vi "Instrument.Temperhum.AppLauncher.vi"(8 "error in":errorcluster, 10 "Config Window":bool, 11 "Debug Mode":bool) -> (0 "error out":errorcluster)   [LabVIEW 2019, in "Instrument.Temperhum.lvclass"]
uses:
  Instrument.Temperhum.lvclass
  <vilib>/JKI/JKI SMO/SMO/Typedefs/SMOState --Enum.ctl
  Instrument UI.Temperhum/Typedefs/Type--enum.ctl
  <userlib>/LevyLab/Instrument Framework/SMOs/Instrument/Instrument.lvclass
  C:/Program Files (x86)/National Instruments/LabVIEW 2019/vi.lib/JKI/JKI SMO/SMO/SMO.lvclass
  <userlib>/LevyLab/Instrument Framework/SMOs/Instrument UI/Instrument UI.lvclass
  C:/Program Files (x86)/National Instruments/LabVIEW 2019/vi.lib/JKI/JKI SMO/SMO.UI/SMO.UI.lvclass
  Instrument UI.Temperhum/Instrument UI.Temperhum.lvclass
  C:/Program Files (x86)/National Instruments/LabVIEW 2019/user.lib/LevyLab/Instrument Framework/SMOs/Instrument UI/Instrument UI.lvclass
  C:/Program Files (x86)/National Instruments/LabVIEW 2019/user.lib/LevyLab/Instrument Framework/SMOs/Instrument/Instrument.lvclass
  <userlib>/LevyLab/Instrument Framework/SMOs/Configuration/Configuration.lvclass
  <vilib>/JKI/JKI SMO/SMO/SMO.lvclass/SMO.ctl
  <userlib>/LevyLab/Instrument Framework/SMOs/Configuration/Configuration.lvclass/Configuration.ctl
  Instrument UI.Temperhum/Typedefs/Instrument UI.Temperhum.UI--Cluster.ctl
  Temperhum.PCSensor/Temperhum.PCSensor.lvclass
  Temperhum.Thorlabs/Temperhum.Thorlabs.lvclass
  <vilib>/JKI/JKI SMO/SMO/Private/ReftoDVR--SMO.vi
  <vilib>/JKI/JKI SMO/SMO/SMO.lvclass
  <vilib>/JKI/JKI SMO/SMO.UI/SMO.UI.lvclass
panel:
  in  "Examine Configuration.ini":bool
  in  "Choose hardware type":T1
  in  "Splash Status":string="Push Start to Start..." caption="String"
  in  "Start Application":bool caption="Play"
  in  "Stop Application":bool caption="Stop"
  out "UI SMO State":T2=enum."Stopped"
  out "SMO State":T2
  # "Example Instrument SMO Test Launcher"
  # "For instructions on how to use the JKI State Machine Objects, examples and video tutorials, visit:\nhttp://jki.net/state-machine-objects/\n\nJKI State Machine Objects™\nhttp://jki.net/state-machine-objects/\nCopyright (C) 2005-2015, JKI <info@jki.net>\nALL RIGHTS RESERVED"
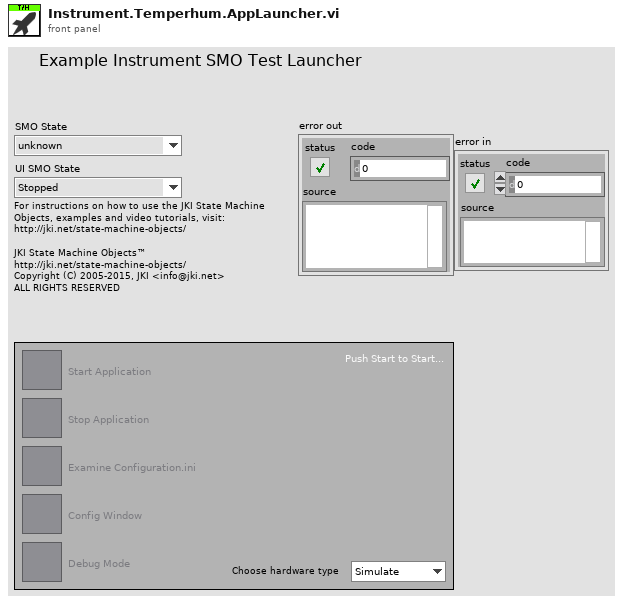
[diagram p1: front panel]
types:
  T1 = typedef "Instrument UI.Temperhum.lvclass/Type--enum.ctl" = enum16{"Simulate", "PCsensor", "Thorlabs"}
  T2 = typedef "SMO.lvclass/SMOState --Enum.ctl" = enum16{"unknown", "Created", "Started", "Stopped"}
  T3 = enum32{"Invalid", "Standard", "Closed", "Hidden", "Minimized", "Maximized"}
  T4 = enum32{"invalid app kind", "Development System", "Run Time System", "Student Edition", "Embedded LabVIEW", "Evaluation", "Custom"}
  T5 = typedef "Instrument UI.Temperhum.lvclass/Instrument UI.Temperhum.UI--Cluster.ctl" = cluster{"HW Type":T1}
  T6 = cluster{"Core":cluster{"Current VI Reference":refnum<vi>, "Close Panel on Exit?":bool}, "Instrument":refnum<class "Instrument.lvclass">, "Instrument UI":refnum<class "Instrument UI.lvclass">, "Configuration":refnum<class "Configuration.lvclass">}
  T7 = cluster{"Current VI Reference":refnum<vi>, "Close Panel on Exit?":bool}
  T8 = typedef "SMO.lvclass/Public Events.ctl" = cluster{"Error":refnum<user-event>, "State":refnum<user-event>, "Reserve State":refnum<user-event>}
  T9 = cluster{"Event Registration Refnum":refnum<event-registration>, "Event Registration Refnum":refnum<event-registration>}
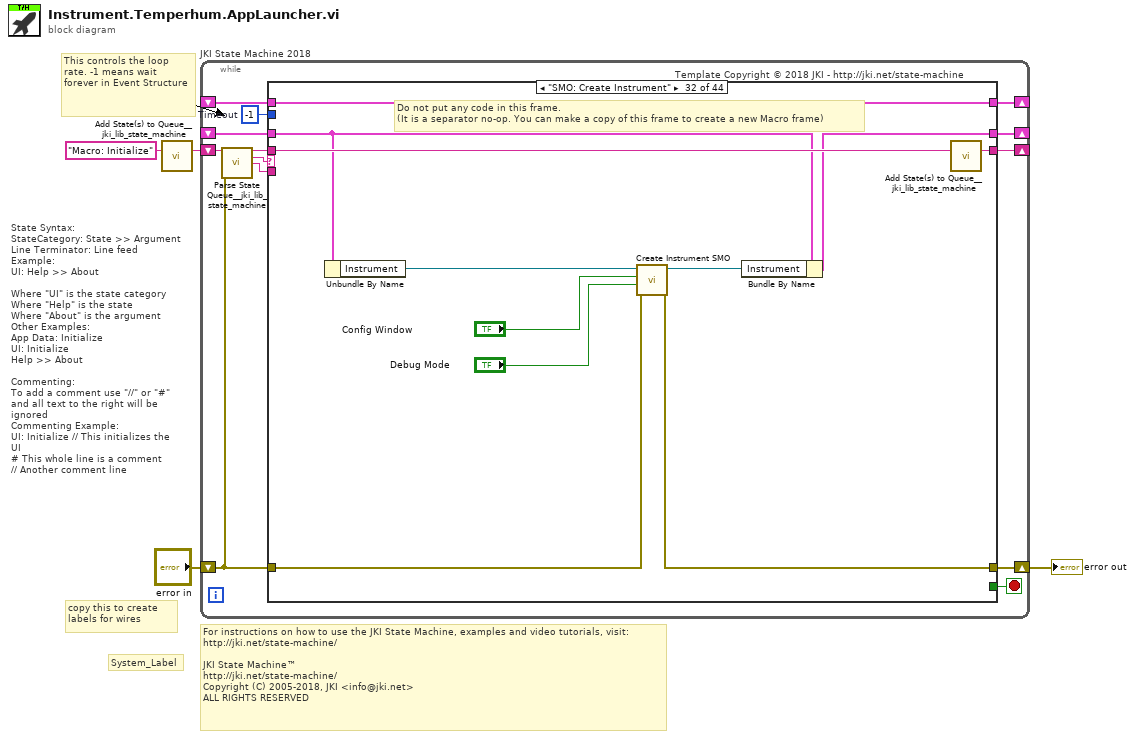
[diagram p0: block diagram]
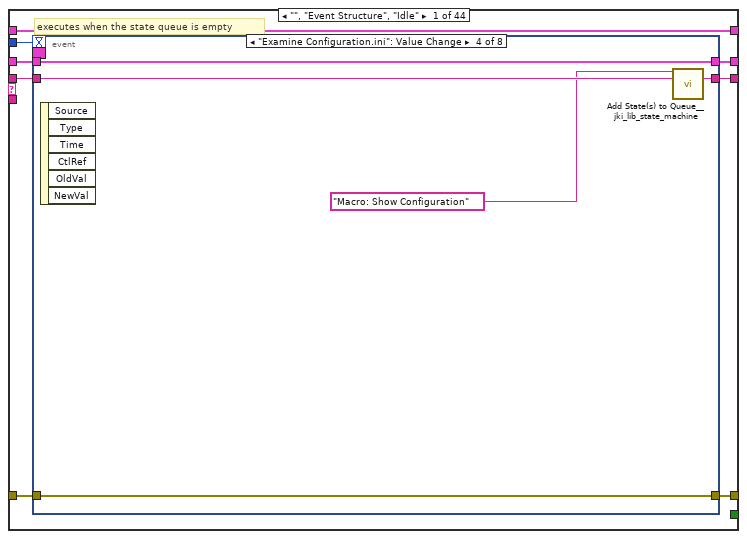
[diagram p2: hidden frame]
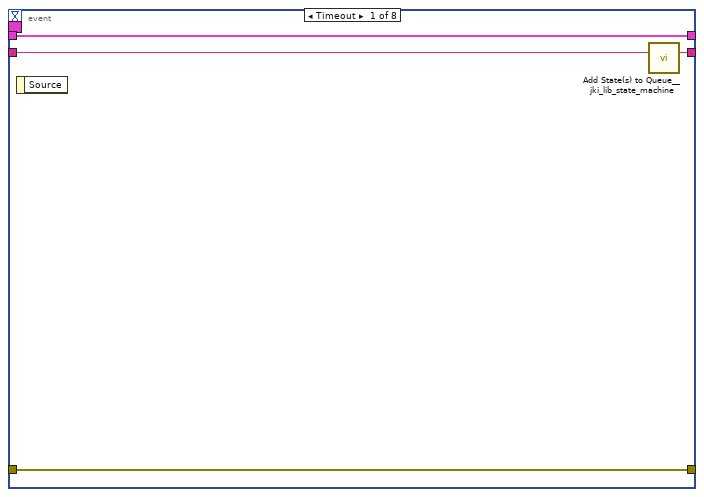
[diagram p3: hidden frame]
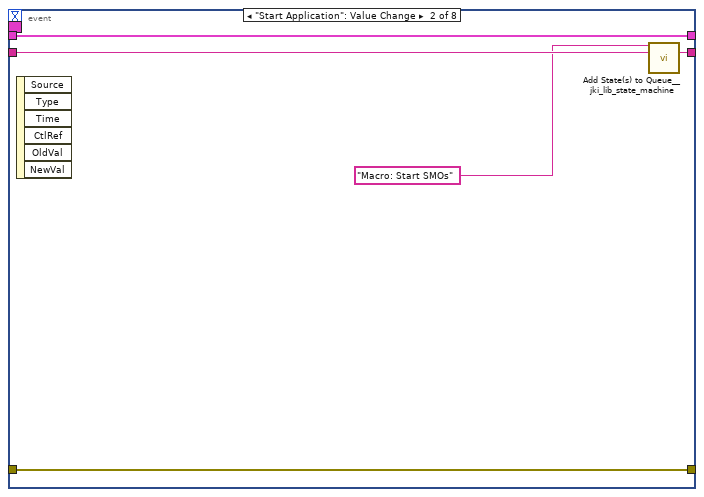
[diagram p4: hidden frame]
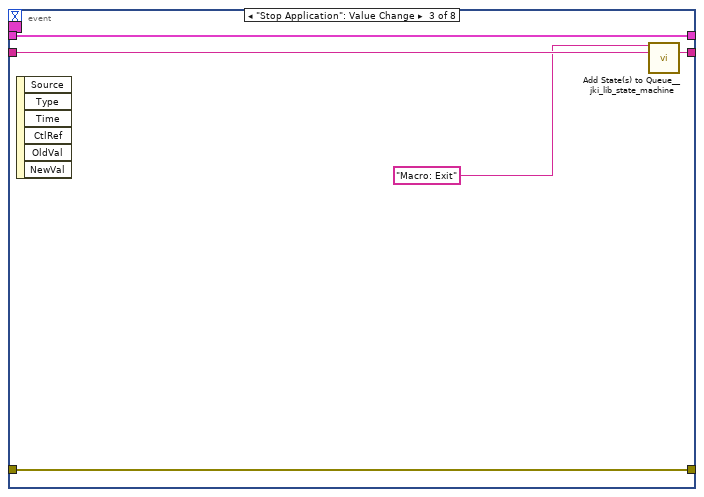
[diagram p5: hidden frame]
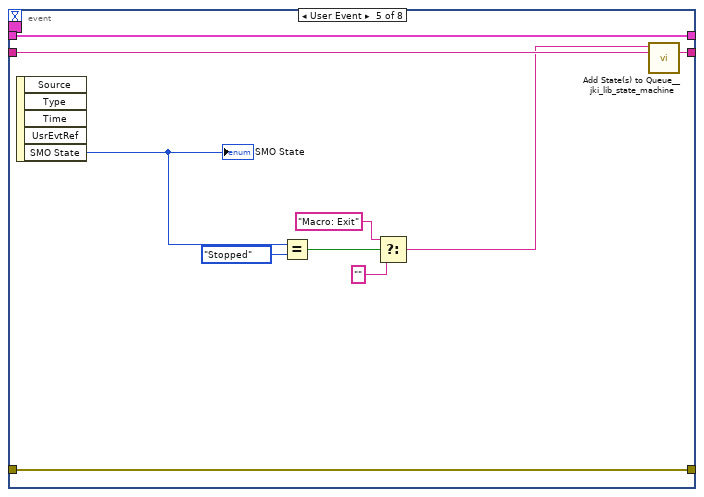
[diagram p6: hidden frame]
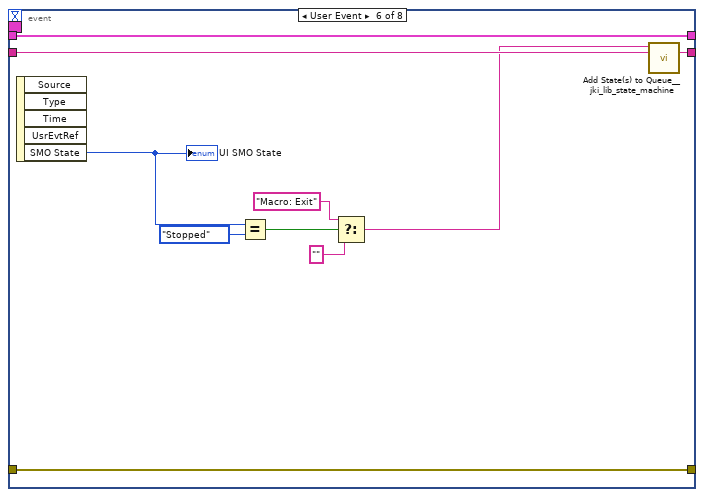
[diagram p7: hidden frame]
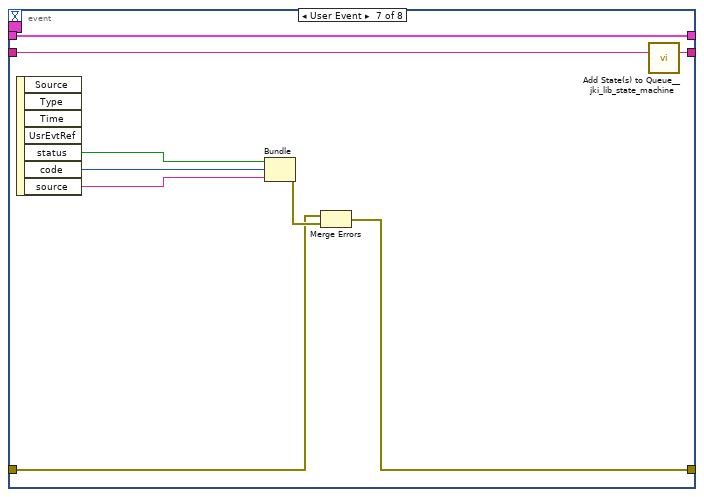
[diagram p8: hidden frame]
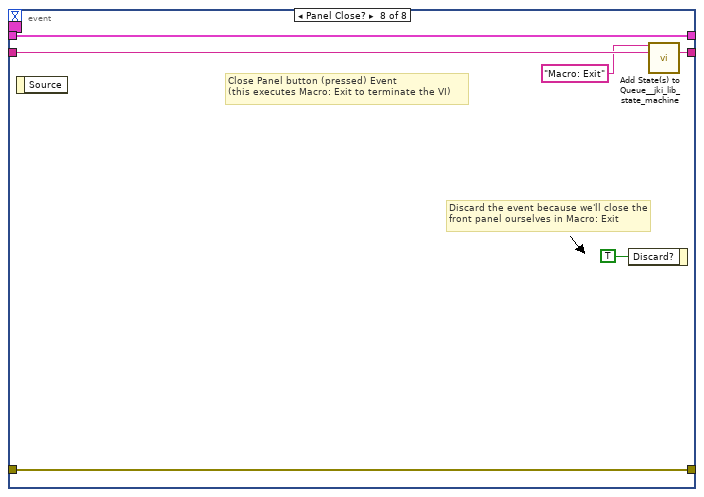
[diagram p9: hidden frame]
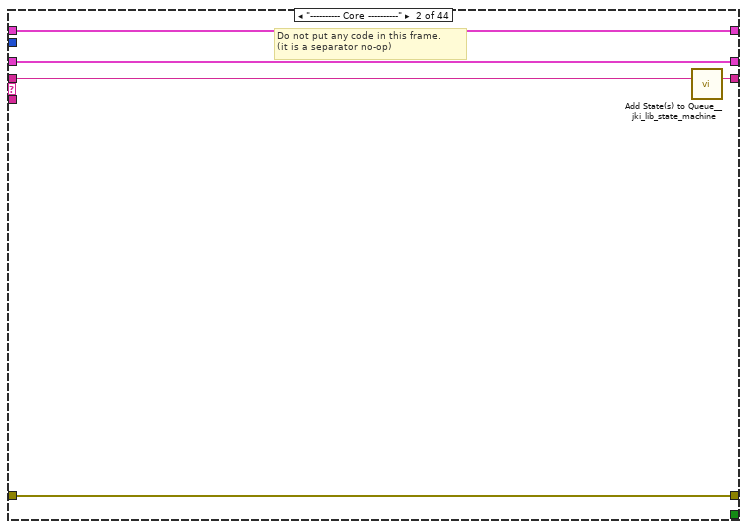
[diagram p10: hidden frame]
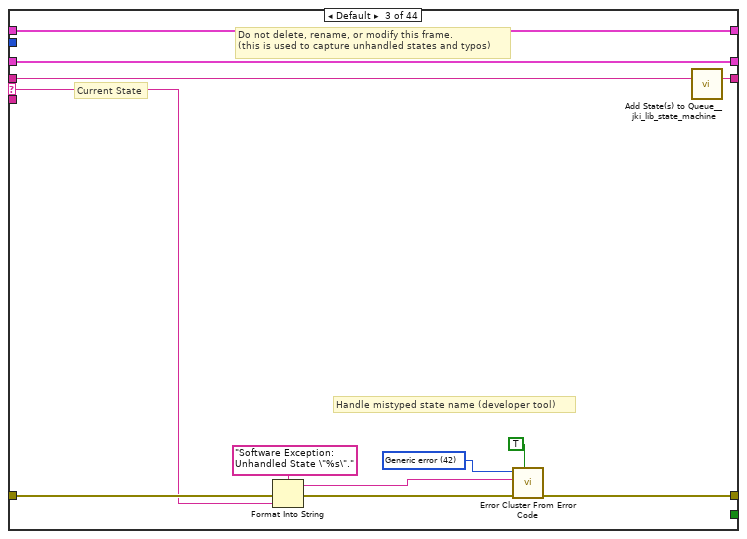
[diagram p11: hidden frame]
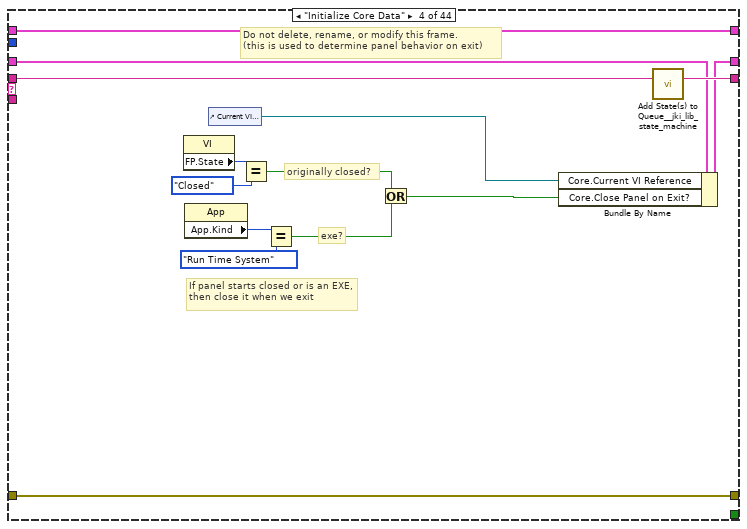
[diagram p12: hidden frame]
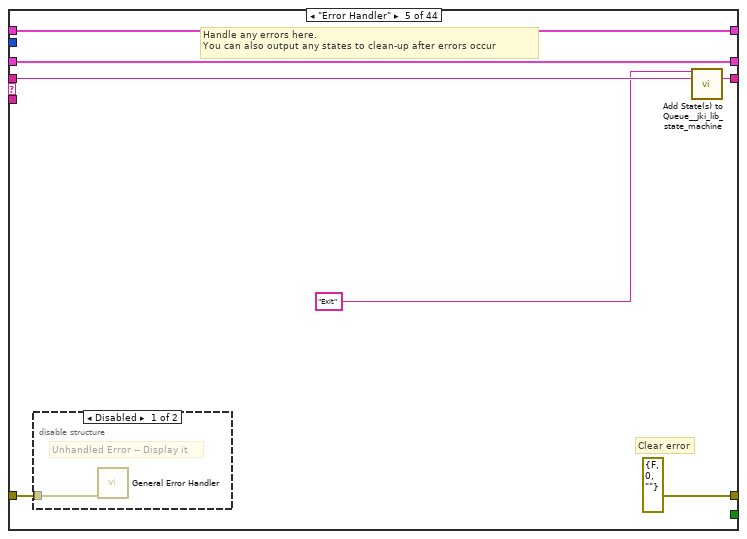
[diagram p13: hidden frame]
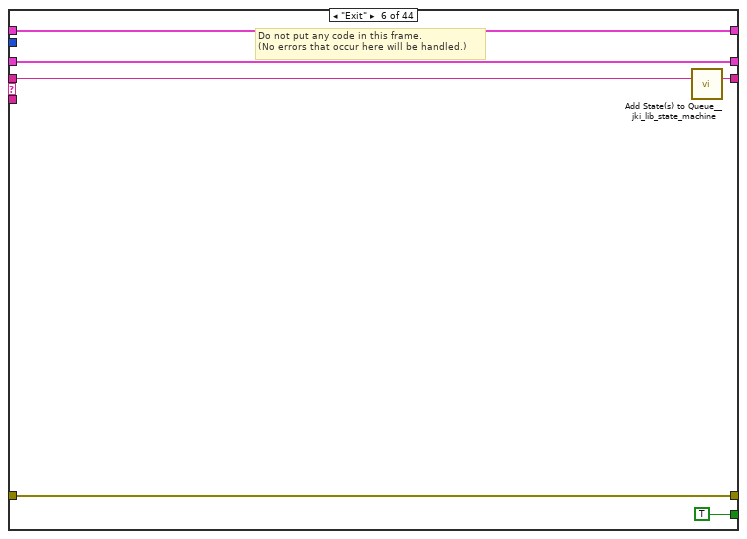
[diagram p15: hidden frame]
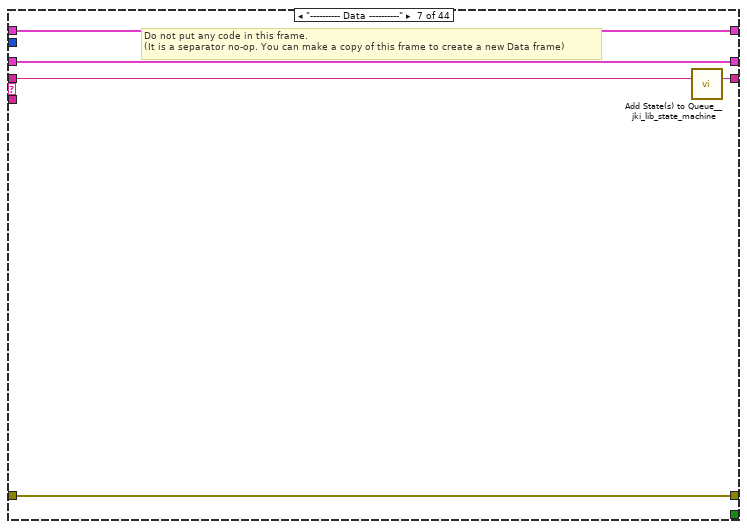
[diagram p16: hidden frame]
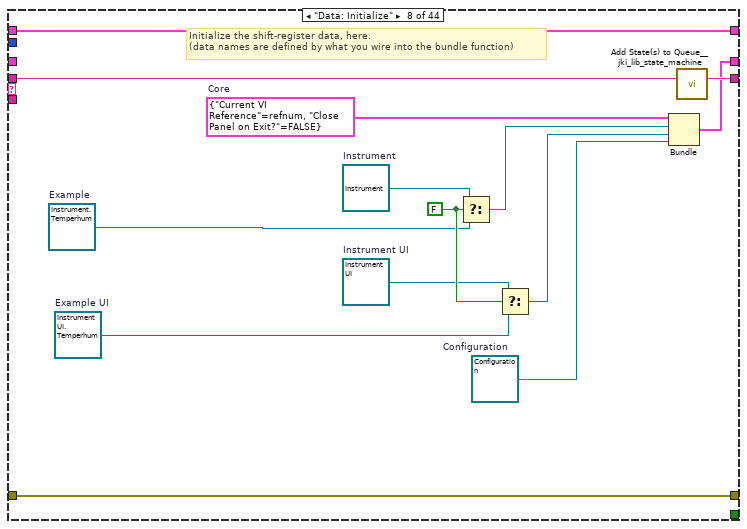
[diagram p17: hidden frame]
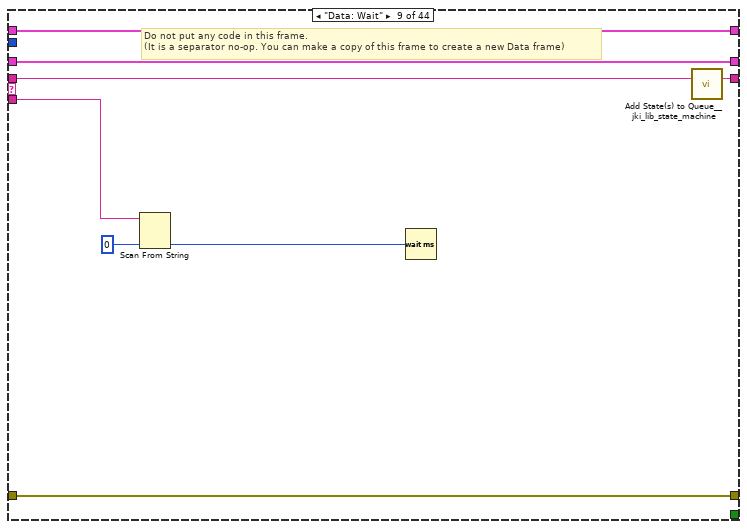
[diagram p18: hidden frame]
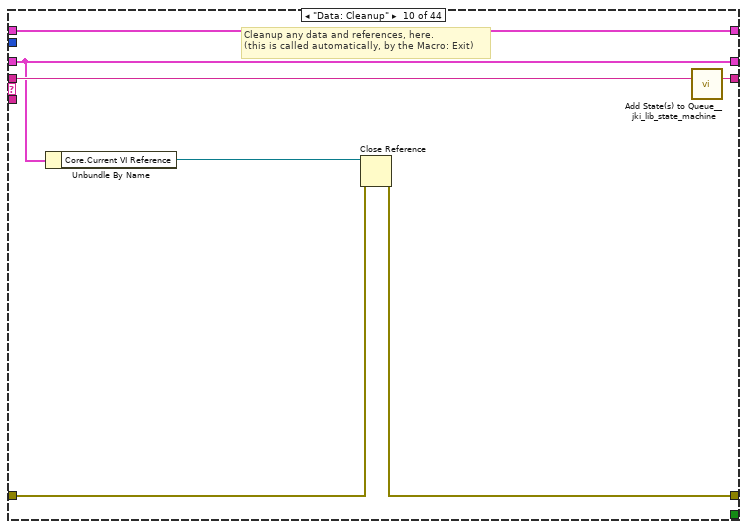
[diagram p19: hidden frame]
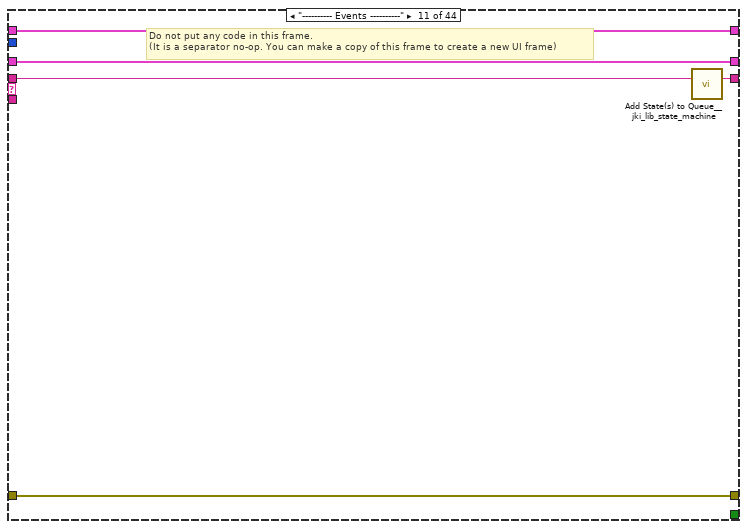
[diagram p20: hidden frame]
diagram:
  # "For instructions on how to use the JKI State Machine, examples and video tutorials, visit:\nhttp://jki.net/state-machine/\n\nJKI State Machine™\nhttp://jki.net/state-machine/\nCopyright (C) 2005-2018, JKI <info@jki.net>\nALL RIGHTS RESERVED"
  # "State Syntax:\nStateCategory: State >> Argument\nLine Terminator: Line feed\nExample:\nUI: Help >> About\n\nWhere \"UI\" is the state category\nWhere \"Help\" is the state\nWhere \"About\" is the argument\nOther Examples:\nApp Data: Initialize\nUI: Initialize\nHelp >> About\n\nCommenting:\nTo add a comment use \"//\" or \"#\" and all text to the right will be ignored\nCommenting Example:\nUI: Initialize // This initializes the UI\n# This whole line is a comment\n// Another comment line"
  # "copy this to create labels for wires"
  # "This controls the loop rate. -1 means wait forever in Event Structure"
  # "System_Label"
  n1 = call <vilib>:"Add State(s) to Queue__jki_lib_state_machine.vi"("State(s) in (\"\")"="Macro: Initialize") -> ("States Out"=w4:string)  [unwired: 14 in]
  n2 = while "JKI State Machine 2018" {
    shift-right: [w11] -> _
    shift-left: _ -> [w6]
    shift-right: [w14] -> w2
    shift-left: "error in" -> [w9]
    shift-right: [w13] -> _
    shift-left: w4 -> [w15]
    shift-right: [w8] -> _
    shift-left: _ -> [w7]
    stop <- w12 stop-if-true
    w10 = -1  # Timeout
    # "Template Copyright © 2018 JKI - http://jki.net/state-machine"
    n3 = call <vilib>:"Parse State Queue__jki_lib_state_machine.vi"("State Queue"=w15, "Error In (no error)"=w9) -> ("Remaining States"=w17:string, "Current State"=w5:string, "Arguments"=w16:string)  [unwired: 11 in]
    n4 = case shown="\"SMO: Create Instrument\"" w5 {
      selector: w5 -> [_ _ w86 _ _ _ _ _ _ _ _ _ _ _ _ _ _ _ _ _ _ _ _ _ _ _ _ _ _ _ _ _ _ _ _ _ _ _ _ _ _ _ _ _]
      tunnel: w17 -> [w25 w84 w90 w110 w117 w124 w129 w143 w151 w158 w163 w176 w182 w187 w193 w200 w212 w290 w297 w309 w321 w335 w340 w345 w351 w357 w363 w369 w381 w386 w395 w409 w418 w428 w435 w446 w461 w476 w491 w506 w521 w530 w537 w542]
      tunnel: w16 -> [_ _ _ _ _ _ _ _ w144 _ _ _ _ _ _ w195 w206 _ _ _ _ _ _ _ _ _ _ _ _ _ _ _ _ _ _ _ _ _ _ _ _ _ w534 _]
      tunnel: [w22 w82 w92 w107 errorcluster {"status"=FALSE, "code"=0, "source"=""} ("error out") w121 w127 w138 w149 w154 w161 w165 w177 w185 w188 w196 w209 w280 w292 w302 w314 w326 w338 w343 w349 w355 w361 w367 w379 w384 w393 w405 w410 w419 w429 w442 w457 w472 w488 w503 w518 w528 w532 w540] -> w14
      tunnel: w9 -> [w21 w82 w91 w107 w113 w121 w127 w138 w149 w155 w161 w167 w178 w185 w190 w197 w210 w281 w291 w301 w313 w322 w338 w343 w349 w355 w361 w367 w379 w384 w393 w406 w411 w420 w430 w439 w453 w469 w486 w501 w514 w528 w533 w540]
      tunnel: [w24 w83 w89 w109 w116 w123 w128 w142 w150 w157 w162 w175 w181 w186 w192 w199 w211 w289 w296 w308 w320 w334 w339 w344 w350 w356 w362 w368 w380 w385 w394 w408 w417 w427 w434 w445 w460 w475 w490 w505 w520 w529 w536 w541] -> w13
      tunnel: [_ _ _ _ _ TRUE _ _ _ _ _ _ _ _ _ _ _ _ _ _ _ _ _ _ _ _ _ _ _ _ _ _ _ _ _ _ _ _ _ _ _ _ _ _] -> w12
      tunnel: [w20 w81 w88 w108 w114 w122 w126 w141 w148 w153 w160 w170 w180 w184 w191 w198 w208 w278 w293 w299 w316 w330 w337 w342 w348 w354 w360 w366 w378 w383 w388 w404 w413 w424 w432 w443 w458 w473 w487 w502 w517 w527 w535 w539] -> w11
      tunnel: w10 -> [w19 _ _ _ _ _ _ _ _ _ _ _ _ _ _ _ _ _ _ _ _ _ _ _ _ _ _ _ _ _ _ _ _ _ _ _ _ _ _ _ _ _ _ _]
      tunnel: [w18 w80 w85 w97 w111 w119 w125 w139 w147 w152 w159 w173 w179 w183 w189 w194 w205 w279 w295 w307 w319 w333 w336 w341 w346 w353 w359 w365 w372 w382 w392 w407 w416 w426 w433 w444 w459 w474 w489 w504 w519 w526 w531 w538] -> w8
      tunnel: w7 -> [w18 w80 w85 w97 w111 w119 w125 w139 w147 w152 w159 _ w179 w183 w189 w194 w205 w279 w295 w307 w319 w333 w336 w341 w346 w353 w359 w365 w372 w382 w392 w407 w416 w426 w433 w444 w459 w474 w489 w504 w519 w526 w531 w538]
      tunnel: w6 -> [w23 w81 w88 w103 w114 w122 w126 _ w148 w153 w160 w170 w180 w184 w191 w198 w208 w278 w293 w298 w315 w329 w337 w342 w348 w354 w360 w366 w378 w383 w389 w402 w414 w425 w432 w443 w458 w473 w487 w502 w517 w527 w535 w539]
      frame "", "Event Structure", "Idle" {
        # "executes when the state queue is empty"
        n5 = event shown="[3] \"Examine Configuration.ini\": Value Change" {
          selector: w18 -> [_ _ _ _ _ _ _ _]
          dyn-events: _ -> [_ _ _ _ _ _ _ _]
          timeout: w19 -> [_ _ _ _ _ _ _ _]
          tunnel: w25 -> [w29 w34 w39 w44 w54 w64 w73 w79]
          tunnel: [w28 w33 w38 w43 w53 w63 w72 w78] -> w24
          tunnel: w23 -> [w26 w31 w36 w41 w51 w61 w71 w76]
          tunnel: [w27 w32 w37 w42 w52 w62 w68 w77] -> w22
          tunnel: w21 -> [w27 w32 w37 w42 w52 w62 w69 w77]
          tunnel: [w26 w31 w36 w41 w51 w61 w71 w76] -> w20
          event Timeout {
            n6 = event-data() -> ()  [unwired: 1 in, 1 out]
            n7 = call <vilib>:"Add State(s) to Queue__jki_lib_state_machine.vi"("State(s) in (\"\")"=w29) -> ("States Out"=w28:string)  [unwired: 14 in]
          }
          event "Start Application": Value Change {
            n8 = event-data() -> ()  [unwired: 1 in, 6 out]
            n9 = call <vilib>:"Add State(s) to Queue__jki_lib_state_machine.vi"("State(s) in Front (\"\")"="Macro: Start SMOs" ("State(s) in Front (\"\")"), "State(s) in (\"\")"=w34) -> ("States Out"=w33:string)  [unwired: 13 in]
          }
          event "Stop Application": Value Change {
            n10 = event-data() -> ()  [unwired: 1 in, 6 out]
            n11 = call <vilib>:"Add State(s) to Queue__jki_lib_state_machine.vi"("State(s) in Front (\"\")"="Macro: Exit" ("State(s) in Front (\"\")"), "State(s) in (\"\")"=w39) -> ("States Out"=w38:string)  [unwired: 13 in]
          }
          event "Examine Configuration.ini": Value Change {
            n12 = event-data() -> ()  [unwired: 1 in, 6 out]
            n13 = call <vilib>:"Add State(s) to Queue__jki_lib_state_machine.vi"("State(s) in Front (\"\")"="Macro: Show Configuration" ("State(s) in Front (\"\")"), "State(s) in (\"\")"=w44) -> ("States Out"=w43:string)  [unwired: 13 in]
          }
          event User Event {
            n14 = event-data() -> ("SMO State"=w46:T2)  [unwired: 1 in, 4 out]
            "SMO State" <- w46
            n15 = Equal?(x=w46, y=SMOState_--Enum."Stopped") -> (x = y?=w49:bool)
            n16 = Select(t="Macro: Exit", s=w49, f="" ("State(s) in Front (\"\")")) -> (s? t:f=w45:string)
            n17 = call <vilib>:"Add State(s) to Queue__jki_lib_state_machine.vi"("State(s) in Front (\"\")"=w45, "State(s) in (\"\")"=w54) -> ("States Out"=w53:string)  [unwired: 13 in]
          }
          event User Event {
            n18 = event-data() -> ("SMO State"=w55:T2)  [unwired: 1 in, 4 out]
            "UI SMO State" <- w55
            n19 = Equal?(x=w55, y=SMOState_--Enum."Stopped") -> (x = y?=w59:bool)
            n20 = Select(t="Macro: Exit", s=w59, f="" ("State(s) in Front (\"\")")) -> (s? t:f=w57:string)
            n21 = call <vilib>:"Add State(s) to Queue__jki_lib_state_machine.vi"("State(s) in Front (\"\")"=w57, "State(s) in (\"\")"=w64) -> ("States Out"=w63:string)  [unwired: 13 in]
          }
          event User Event {
            n22 = event-data() -> ("status"=w65:bool, "code"=w67:i32, "source"=w66:string)  [unwired: 1 in, 4 out]
            n23 = Bundle("status"=w65, "code"=w67, "source"=w66) -> (w70:errorcluster)  [unwired: 1 in]
            n24 = Merge Errors(w69, w70) -> (w68:errorcluster)
            n25 = call <vilib>:"Add State(s) to Queue__jki_lib_state_machine.vi"("State(s) in (\"\")"=w73) -> ("States Out"=w72:string)  [unwired: 14 in]
          }
          event Panel Close? {
            # "Discard the event because we'll close the front panel ourselves in Macro: Exit"
            # "Close Panel button (pressed) Event\n(this executes Macro: Exit to terminate the VI)"
            n26 = event-data() -> ()  [unwired: 1 in, 1 out]
            n27 = event-data("Discard?"=TRUE) -> ()  [unwired: 1 in, 1 out]
            n28 = call <vilib>:"Add State(s) to Queue__jki_lib_state_machine.vi"("State(s) in Front (\"\")"="Macro: Exit", "State(s) in (\"\")"=w79) -> ("States Out"=w78:string)  [unwired: 13 in]
          }
        }
      }
      frame "---------- Core ----------" {
        # "Do not put any code in this frame.\n(it is a separator no-op)"
        n29 = call <vilib>:"Add State(s) to Queue__jki_lib_state_machine.vi"("State(s) in (\"\")"=w84) -> ("States Out"=w83:string)  [unwired: 14 in]
      }
      frame Default {
        w95 = 42 items=["No error", "Argument error", "Memory is full", "Out of zone", "End of file", "File already open", "Generic file I/O error", "File not found", "File permission error", "Disk is full", "Duplicate path", "Too many files open", "System feature not enabled", "Resource file not found", "Cannot add resource", "Resource not found", "Image not found", "Image memory error", "Pen does not exist", "Config type invalid", "Config token not found", "Config parse error", "Config memory error", "Bad external code format", "Bad external code offset", "External code not present", "Null window", "Destroy window error", "Null menu", "Print aborted", "Bad print record", "Print driver error", "Windows error during printing", "Memory error during printing", "Print dialog error", "Generic print error", "Invalid device refnum", "Device not found", "Device parameter error", "Device unit error", "Cannot open device", "Device call aborted", "Generic error", "Cancelled by user", "Object ID too low", "Object ID too high", "Object not in heap", "Unknown heap", "Unknown object (invalid DefProc)", "Unknown object (DefProc not in table)", "Message out of range", "Invalid (null) method", "Unknown message", "Manager call not supported", "Bad address", "Network operation in progress", "Network operation timed out", "Connection is busy", "Network attribute not supported", "Network error", "Address in use", "System out of memory", "Connection aborted", "Connection refused", "Not connected", "Already connected", "Connection closed", "Initialization error (interapplication manager)", "Bad occurrence", "Wait on unbound occurrence handler", "Occurrence queue overflow", "Datalog type conflict", "Unused", "Unrecognized type (interapplication manager)", "Memory corrupt", "Failed to make temporary DLL", "Old CIN version", "Drag socket not found", "Failed to load drop-object", "Failed to register OLE object", "Failed to release OLE object", "Format specifier type mismatch", "Unknown format specifier", "Too few format specifiers", "Too many format specifiers", "Scan failed", "Newer CIN version", "Error converting to variant", "Runtime menu error", "Password tampered", "Variant attribute not found", "Incompatible variant data type", "Event data is not available", "Event Store is not present", "Occurrence is not found", "Event Queue is not created", "Event info is not available", "Refnum passed is NULL", "Error retrieving Class GUID", "Error retrieving CoClass GUID", "Error retrieving TypeLib GUID.", "Bad built application magic bytes.", "Specific driver is different from the specific driver associated with the Logical Name.", "There is no session opened to the class driver.", "Max Error", "MAX - Error with config objects", "MAX - Error loading configuration", "MAX - Group not supported"]
        # "Current State"
        # "Do not delete, rename, or modify this frame.\n(this is used to capture unhandled states and typos)"
        # "Handle mistyped state name (developer tool)"
        n30 = Format Into String(format string="Software Exception: Unhandled State \"%s\"." ("message"), error in=w91, w86) -> (resulting string=w94:string, error out=w93:errorcluster)  [unwired: 1 in]
        n31 = call <vilib>:"Error Cluster From Error Code.vi"("show call chain? (False)"=TRUE, "error in (no error)"=w93, "error message (\"\")"=w94, "error code (0)"=w95) -> ("error out"=w92:errorcluster)  [unwired: 5 in]
        n32 = call <vilib>:"Add State(s) to Queue__jki_lib_state_machine.vi"("State(s) in (\"\")"=w90) -> ("States Out"=w89:string)  [unwired: 14 in]
      }
      frame "Initialize Core Data" {
        # "Do not delete, rename, or modify this frame.\n(this is used to determine panel behavior on exit)"
        # "originally closed?"
        # "exe?"
        # "If panel starts closed or is an EXE, then close it when we exit"
        n33 = property class="VI"() -> ("FP.State"=w100:T3)  [unwired: 2 in, 2 out]
        n34 = property class="App"() -> ("App.Kind"=w106:T4)  [unwired: 2 in, 2 out]
        n35 = control-ref of="Current VI Reference"() -> (w101:refnum<vi>)
        n36 = Equal?(x=w100, y=T3."Closed" ("Front Panel Window:State")) -> (x = y?=w98:bool)
        n37 = Equal?(x=w106, y=T4."Run Time System" ("Application:Kind")) -> (x = y?=w104:bool)
        n38 = Or(x=w98, y=w104) -> (x .or. y?=w102:bool)
        n39 = Bundle By Name(cluster=w103, "Core.Current VI Reference"=w101, "Core.Close Panel on Exit?"=w102) -> (w108:T6)
        n40 = call <vilib>:"Add State(s) to Queue__jki_lib_state_machine.vi"("State(s) in (\"\")"=w110) -> ("States Out"=w109:string)  [unwired: 14 in]
      }
      frame "Error Handler" {
        # "Handle any errors here.\nYou can also output any states to clean-up after errors occur"
        # "Clear error"
        n41 = disable-structure shown="Disabled" {
          disable-tunnel: w113 -> [w118 _]
          frame Disabled {
            # "Unhandled Error -- Display it"
            n42 = call <vilib>:"General Error Handler.vi"("error in (no error)"=w118) -> ()  [unwired: 10 in, 5 out]
          }
          frame Enabled {
          }
        }
        n43 = call <vilib>:"Add State(s) to Queue__jki_lib_state_machine.vi"("State(s) in Front (\"\")"="Exit", "State(s) in (\"\")"=w117) -> ("States Out"=w116:string)  [unwired: 13 in]
      }
      frame "Exit" {
        # "Do not put any code in this frame.\n(No errors that occur here will be handled.)"
        n44 = call <vilib>:"Add State(s) to Queue__jki_lib_state_machine.vi"("State(s) in (\"\")"=w124) -> ("States Out"=w123:string)  [unwired: 14 in]
      }
      frame "---------- Data ----------" {
        # "Do not put any code in this frame.\n(It is a separator no-op. You can make a copy of this frame to create a new Data frame)"
        n45 = call <vilib>:"Add State(s) to Queue__jki_lib_state_machine.vi"("State(s) in (\"\")"=w129) -> ("States Out"=w128:string)  [unwired: 14 in]
      }
      frame "Data: Initialize" {
        w130 = refnum<class "Configuration.lvclass"> refnum  # Configuration
        w134 = FALSE ("s")
        w133 = refnum<class "Instrument.Temperhum.lvclass"> refnum  # Example
        w132 = refnum<class "Instrument UI.Temperhum.lvclass"> refnum  # Example UI
        w131 = refnum<class "Instrument UI.lvclass"> refnum  # Instrument UI
        w137 = refnum<class "Instrument.lvclass"> refnum  # Instrument
        w140 = T7 {"Current VI Reference"=refnum, "Close Panel on Exit?"=FALSE}  # Core
        # "Initialize the shift-register data, here.\n(data names are defined by what you wire into the bundle function)"
        n46 = Select(t=w137, s=w134, f=w133) -> (s? t:f=w136:refnum<class "Instrument.lvclass">)
        n47 = Select(t=w131, s=w134, f=w132) -> (s? t:f=w135:refnum<class "Instrument UI.lvclass">)
        n48 = Bundle("Core"=w140, "Instrument"=w136, "Instrument UI"=w135, "Configuration"=w130) -> (w141:T6)  [unwired: 1 in]
        n49 = call <vilib>:"Add State(s) to Queue__jki_lib_state_machine.vi"("State(s) in (\"\")"=w143) -> ("States Out"=w142:string)  [unwired: 14 in]
      }
      frame "Data: Wait" {
        # "Do not put any code in this frame.\n(It is a separator no-op. You can make a copy of this frame to create a new Data frame)"
        n50 = Scan From String(input string=w144, default 1=u32 0) -> (output 1=w145:u32)  [unwired: 3 in, 3 out]
        n51 = Wait (ms)(milliseconds to wait=w145) -> ()  [unwired: 1 out]
        n52 = call <vilib>:"Add State(s) to Queue__jki_lib_state_machine.vi"("State(s) in (\"\")"=w151) -> ("States Out"=w150:string)  [unwired: 14 in]
      }
      frame "Data: Cleanup" {
        # "Cleanup any data and references, here.\n(this is called automatically, by the Macro: Exit)"
        n53 = Unbundle By Name(w153) -> ("Core.Current VI Reference"=w156:refnum<vi>)
        n54 = Close Reference(reference=w156, error in (no error)=w155) -> (error out=w154:errorcluster)
        n55 = call <vilib>:"Add State(s) to Queue__jki_lib_state_machine.vi"("State(s) in (\"\")"=w158) -> ("States Out"=w157:string)  [unwired: 14 in]
      }
      frame "---------- Events ----------" {
        # "Do not put any code in this frame.\n(It is a separator no-op. You can make a copy of this frame to create a new UI frame)"
        n56 = call <vilib>:"Add State(s) to Queue__jki_lib_state_machine.vi"("State(s) in (\"\")"=w163) -> ("States Out"=w162:string)  [unwired: 14 in]
      }
      frame "Events: Register" {
        # "Do not put any code in this frame.\n(It is a separator no-op. You can make a copy of this frame to create a new UI frame)"
        n57 = Unbundle By Name(w170) -> ("Instrument"=w169:refnum<class "Instrument.lvclass">, "Instrument UI"=w168:refnum<class "Instrument UI.lvclass">)
        n58 = call <vilib>:"GetPublicEvents.vi"("error in (no error)"=w167, "SMO"=w169) -> ("error out"=w166:errorcluster, "Public Events"=w171:T8)  [unwired: 7 in, 1 out]
        n59 = call <vilib>:"GetPublicEvents.vi"("error in (no error)"=w166, "SMO"=w168) -> ("error out"=w165:errorcluster, "Public Events"=w172:T8)  [unwired: 7 in, 1 out]
        n60 = register-events(w171) -> (reference out=w174:refnum<event-registration>)  [unwired: 2 in, 1 out]
        n61 = register-events(w172) -> (reference out=w164:refnum<event-registration>)  [unwired: 2 in, 1 out]
        n62 = Bundle("Event Registration Refnum"=w174, "Event Registration Refnum"=w164) -> (w173:T9)  [unwired: 1 in]
        n63 = call <vilib>:"Add State(s) to Queue__jki_lib_state_machine.vi"("State(s) in (\"\")"=w176) -> ("States Out"=w175:string)  [unwired: 14 in]
      }
      frame "Events: Unregister" {
        # "Do not put any code in this frame.\n(It is a separator no-op. You can make a copy of this frame to create a new UI frame)"
        n64 = Unregister For Events(event registration refnum=w179, error in=w178) -> (error out=w177:errorcluster)
        n65 = call <vilib>:"Add State(s) to Queue__jki_lib_state_machine.vi"("State(s) in (\"\")"=w182) -> ("States Out"=w181:string)  [unwired: 14 in]
      }
      frame "---------- UI ----------" {
        # "Do not put any code in this frame.\n(It is a separator no-op. You can make a copy of this frame to create a new UI frame)"
        n66 = call <vilib>:"Add State(s) to Queue__jki_lib_state_machine.vi"("State(s) in (\"\")"=w187) -> ("States Out"=w186:string)  [unwired: 14 in]
      }
      frame "UI: Initialize" {
        # "Initialize the User Interface, here.\n(this is called automatically, by the Macro: Init)"
        n67 = invoke on="Stop Application" class="Bool" method="Reinit To Default"() -> ()  [unwired: 3 in, 3 out]
        n68 = invoke on="error out" class="Clust (strict)" method="Reinit To Default"() -> ()  [unwired: 3 in, 3 out]
        n69 = invoke on="SMO State 2" class="Enum (strict)" method="Reinit To Default"() -> ()  [unwired: 3 in, 3 out]
        n70 = invoke on="Start Application" class="Bool" method="Reinit To Default"() -> ()  [unwired: 3 in, 3 out]
        n71 = call <userlib>:"Fit VI window to Largest Dec__ogtk.vi"("error in (no error)"=w190) -> ("error out"=w188:errorcluster)  [unwired: 5 in, 1 out]
        n72 = call <vilib>:"Add State(s) to Queue__jki_lib_state_machine.vi"("State(s) in (\"\")"=w193) -> ("States Out"=w192:string)  [unwired: 14 in]
      }
      frame "UI: Cursor Set" {
        # "Argument"
        # "Set and Unset Cursor Busy.\n(Usage: \"UI: Cursor Set >> Busy|Idle\")"
        n73 = case shown="\"Busy\"" w195 {
          tunnel: w197 -> [w202 w204]
          tunnel: [w201 w203] -> w196
          frame "Idle", Default {
            n74 = call <vilib>:"Unset Busy.vi"("error in (no error)"=w202) -> ("error out"=w201:errorcluster)  [unwired: 10 in]
          }
          frame "Busy" {
            n75 = call <vilib>:"Set Busy.vi"("error in (no error)"=w204) -> ("error out"=w203:errorcluster)  [unwired: 9 in, 1 out]
          }
        }
        n76 = call <vilib>:"Add State(s) to Queue__jki_lib_state_machine.vi"("State(s) in (\"\")"=w200) -> ("States Out"=w199:string)  [unwired: 14 in]
      }
      frame "UI: Front Panel State" {
        # "Argument"
        # "Set Front Panel Open or Closed\n(Usage: \"UI: Front Panel State >> Open|Close\")"
        n77 = Unbundle By Name(w208) -> ("Core.Current VI Reference"=w207:refnum<vi>)
        n78 = case shown="\"Open\", \"Standard\", Default" w206 {
          tunnel: w210 -> [w218 w233 w244 w257 w270]
          tunnel: [w220 w234 w246 w259 w272] -> w209
          tunnel: w207 -> [w219 w231 w245 w258 w271]
          frame "Open", "Standard", Default {
            w213 = T3."Standard" ("State")
            n79 = property class="VI"(reference=w219, error in=w218) -> (reference out=w216:refnum<vi>, error out=w217:errorcluster, "FP.State"=w215:T3)
            n80 = Not Equal?(x=w215, y=w213) -> (x != y?=w214:bool)
            n81 = case shown="False" w214 {
              tunnel: [w224 w226] -> w220
              tunnel: w217 -> [w223 w226]
              tunnel: w216 -> [w222 _]
              tunnel: w213 -> [w221 _]
              frame True {
                n82 = invoke class="VI" method="FP.Open"(reference=w222, error in=w223, "Activate"=TRUE, "State"=w221) -> (error out=w224:errorcluster)  [unwired: 1 in, 4 out]
              }
              frame False {
              }
            }
          }
          frame "Close", "Closed" {
            n83 = property class="VI"(reference=w231, error in=w233) -> (reference out=w230:refnum<vi>, error out=w232:errorcluster, "FP.State"=w228:T3)
            n84 = Not Equal?(x=w228, y=T3."Closed" ("Front Panel Window:State")) -> (x != y?=w227:bool)
            n85 = case shown="True" w227 {
              tunnel: [w235 w238] -> w234
              tunnel: w232 -> [w235 w237]
              tunnel: w230 -> [_ w236]
              frame False {
              }
              frame True {
                n86 = invoke class="VI" method="FP.Close"(reference=w236, error in=w237) -> (error out=w238:errorcluster)  [unwired: 1 in, 2 out]
              }
            }
          }
          frame "Hidden", "Hide" {
            w239 = T3."Hidden" ("State")
            n87 = property class="VI"(reference=w245, error in=w244) -> (reference out=w242:refnum<vi>, error out=w243:errorcluster, "FP.State"=w241:T3)
            n88 = Not Equal?(x=w241, y=w239) -> (x != y?=w240:bool)
            n89 = case shown="True" w240 {
              tunnel: [w250 w251] -> w246
              tunnel: w243 -> [w249 w251]
              tunnel: w242 -> [w248 _]
              tunnel: w239 -> [w247 _]
              frame True {
                n90 = invoke class="VI" method="FP.Open"(reference=w248, error in=w249, "State"=w247) -> (error out=w250:errorcluster)  [unwired: 2 in, 4 out]
              }
              frame False {
              }
            }
          }
          frame "Minimize", "Minimized" {
            w252 = T3."Minimized" ("State")
            n91 = property class="VI"(reference=w258, error in=w257) -> (reference out=w255:refnum<vi>, error out=w256:errorcluster, "FP.State"=w254:T3)
            n92 = Not Equal?(x=w254, y=w252) -> (x != y?=w253:bool)
            n93 = case shown="True" w253 {
              tunnel: [w263 w264] -> w259
              tunnel: w256 -> [w262 w264]
              tunnel: w255 -> [w261 _]
              tunnel: w252 -> [w260 _]
              frame True {
                n94 = invoke class="VI" method="FP.Open"(reference=w261, error in=w262, "State"=w260) -> (error out=w263:errorcluster)  [unwired: 2 in, 4 out]
              }
              frame False {
              }
            }
          }
          frame "Maximize", "Maximized" {
            w265 = T3."Maximized" ("State")
            n95 = property class="VI"(reference=w271, error in=w270) -> (reference out=w268:refnum<vi>, error out=w269:errorcluster, "FP.State"=w267:T3)
            n96 = Not Equal?(x=w267, y=w265) -> (x != y?=w266:bool)
            n97 = case shown="True" w266 {
              tunnel: [w276 w277] -> w272
              tunnel: w269 -> [w275 w277]
              tunnel: w268 -> [w274 _]
              tunnel: w265 -> [w273 _]
              frame True {
                n98 = invoke class="VI" method="FP.Open"(reference=w274, error in=w275, "State"=w273) -> (error out=w276:errorcluster)  [unwired: 2 in, 4 out]
              }
              frame False {
              }
            }
          }
        }
        n99 = call <vilib>:"Add State(s) to Queue__jki_lib_state_machine.vi"("State(s) in (\"\")"=w212) -> ("States Out"=w211:string)  [unwired: 14 in]
      }
      frame "UI: Set Background Color" {
        # "Do not put any code in this frame.\n(It is a separator no-op. You can make a copy of this frame to create a new UI frame)"
        n100 = property class="VI"(error in=w281) -> (error out=w283:errorcluster, "Panel"=w284:refnum<vi>)  [unwired: 1 in, 1 out]
        n101 = property class="Pnl"(reference=w284, error in=w283) -> (error out=w282:errorcluster, "Panes[]"=w285:refnum<vi>[])  [unwired: 1 out]
        n102 = Index Array(array=w285, index=0) -> (element=w287:refnum<vi>)
        n103 = property class="Pane"(reference=w287, error in=w282, "PaneColor"=u32 16777238 ("Color Box")) -> (error out=w280:errorcluster)  [unwired: 1 out]
        n104 = call <vilib>:"Add State(s) to Queue__jki_lib_state_machine.vi"("State(s) in (\"\")"=w290) -> ("States Out"=w289:string)  [unwired: 14 in]
      }
      frame "UI: Open Configuration.ini" {
        # "Do not put any code in this frame.\n(It is a separator no-op. You can make a copy of this frame to create a new UI frame)"
        n105 = Unbundle By Name(w293) -> ("Instrument"=w294:refnum<class "Instrument.lvclass">)
        n106 = call <userlib>:"Examine Configuration.vi"("error in (no error)"=w291, "Instrument in"=w294) -> ("error out"=w292:errorcluster)  [unwired: 8 in, 1 out]
        n107 = call <vilib>:"Add State(s) to Queue__jki_lib_state_machine.vi"("State(s) in (\"\")"=w297) -> ("States Out"=w296:string)  [unwired: 14 in]
      }
      frame "UI: Init UI Config" {
        # "Do not put any code in this frame.\n(It is a separator no-op. You can make a copy of this frame to create a new UI frame)"
        n108 = call <userlib>:"Default Path.vi"("error in (no error)"=w301, "Folder Name [Application Name]"="TemperHum" ("Folder Name")) -> ("error out"=w303:errorcluster, "Configuration out"=w305:refnum<class "Configuration.lvclass">)  [unwired: 8 in]
        n109 = call <userlib>:"Write Section.vi"("error in (no error)"=w303, "Section"="UI Config", "Configuration in"=w305) -> ("error out"=w302:errorcluster, "Configuration out"=w300:refnum<class "Configuration.lvclass">)  [unwired: 7 in]
        n110 = Bundle By Name(cluster=w298, "Configuration"=w300) -> (w299:T6)
        n111 = call <vilib>:"Add State(s) to Queue__jki_lib_state_machine.vi"("State(s) in (\"\")"=w309) -> ("States Out"=w308:string)  [unwired: 14 in]
      }
      frame "UI: Write UI Config" {
        # "read front panel control"
        # "Do not put any code in this frame.\n(It is a separator no-op. You can make a copy of this frame to create a new UI frame)"
        n112 = local read "Choose hardware type"() -> (w310:T1)
        n113 = Unbundle By Name(w315) -> ("Configuration"=w318:refnum<class "Configuration.lvclass">)
        n114 = Bundle By Name(cluster=T5 {"HW Type"=enum."Simulate"} ("UI"), "HW Type"=w310) -> (w311:T5)
        n115 = call <userlib>:"Write Configuration.vi"("error in (no error)"=w313, "Variant"=w311, "Configuration in"=w318) -> ("error out"=w314:errorcluster, "Configuration out"=w317:refnum<class "Configuration.lvclass">)  [unwired: 7 in]
        n116 = Bundle By Name(cluster=w315, "Configuration"=w317) -> (w316:T6)
        n117 = call <vilib>:"Add State(s) to Queue__jki_lib_state_machine.vi"("State(s) in (\"\")"=w321) -> ("States Out"=w320:string)  [unwired: 14 in]
      }
      frame "UI: Read UI Config" {
        w328 = T5 {"HW Type"=enum."Simulate"} ("UI")
        # "Do not put any code in this frame.\n(It is a separator no-op. You can make a copy of this frame to create a new UI frame)"
        n118 = Unbundle By Name(w329) -> ("Configuration"=w332:refnum<class "Configuration.lvclass">)
        n119 = call <userlib>:"Read Configuration.vi"("INI Fomatted Cluster Type"=w328, "error in (no error)"=w322, "Configuration in"=w332) -> ("error out"=w325:errorcluster, "Configuration"=w331:variant, "Configuration out"=w327:refnum<class "Configuration.lvclass">)  [unwired: 6 in]
        n120 = Variant To Data(error in=w325, type=w328, Variant=w331) -> (data=w324:T5, error out=w326:errorcluster)
        n121 = Unbundle By Name(w324) -> ("HW Type"=w323:T1)
        n122 = local write "Choose hardware type"(w323) -> ()
        n123 = Bundle By Name(cluster=w329, "Configuration"=w327) -> (w330:T6)
        n124 = call <vilib>:"Add State(s) to Queue__jki_lib_state_machine.vi"("State(s) in (\"\")"=w335) -> ("States Out"=w334:string)  [unwired: 14 in]
      }
      frame "UI: Exit" {
        # "Do not put any code in this frame.\n(It is a separator no-op. You can make a copy of this frame to create a new UI frame)"
        n125 = invoke on="Start Application" class="Bool" method="Reinit To Default"() -> ()  [unwired: 3 in, 3 out]
        n126 = invoke on="Stop Application" class="Bool" method="Reinit To Default"() -> ()  [unwired: 3 in, 3 out]
        n127 = call <vilib>:"Add State(s) to Queue__jki_lib_state_machine.vi"("State(s) in (\"\")"=w340) -> ("States Out"=w339:string)  [unwired: 14 in]
      }
      frame "---------- Macro ----------" {
        # "Do not put any code in this frame.\n(It is a separator no-op. You can make a copy of this frame to create a new Macro frame)"
        n128 = call <vilib>:"Add State(s) to Queue__jki_lib_state_machine.vi"("State(s) in (\"\")"=w345) -> ("States Out"=w344:string)  [unwired: 14 in]
      }
      frame "Macro: Initialize" {
        # "Initialization Macro\n(This is called once, when the VI starts)"
        n129 = call <vilib>:"Add State(s) to Queue__jki_lib_state_machine.vi"("State(s) in Front (\"\")"="Data: Initialize\nInitialize Core Data\n//Events: Register\n\nUI: Initialize\nUI: Front Panel State >> Open\n\nUI: Init UI Config\nUI: Read UI Config\n\nUI: Set Background Color\nSplash: Set Status >> ...", "State(s) in (\"\")"=w351) -> ("States Out"=w350:string)  [unwired: 13 in]
      }
      frame "Macro: Show Configuration" {
        # "Do not put any code in this frame.\n(It is a separator no-op. You can make a copy of this frame to create a new Macro frame)"
        n130 = call <vilib>:"Add State(s) to Queue__jki_lib_state_machine.vi"("State(s) in Front (\"\")"="Splash: Set Status >> Opening Configuration...\nUI: Open Configuration.ini\nData: Wait >> 1000\nSplash: Set Status >> ...", "State(s) in (\"\")"=w357) -> ("States Out"=w356:string)  [unwired: 13 in]
      }
      frame "Macro: Start SMOs" {
        (unwired) "Splash: Set Status >> Starting Instrument...\nSMO: Init Class\nSMO: Create Instrument\nSMO: Create Instrument UI\nEvents: Register\nSMO: Start Instrument\nSplash: Set Status >> Instrument Process Started...\nSplash: Set Status >> Starting User Interface...\nSMO: Start Instrument UI\nUI: Front Panel State >> Hide\nSMO: Show Instrument UI" ("State(s) in Front (\"\")")
        # "Do not put any code in this frame.\n(It is a separator no-op. You can make a copy of this frame to create a new Macro frame)"
        n131 = call <vilib>:"Add State(s) to Queue__jki_lib_state_machine.vi"("State(s) in Front (\"\")"="Splash: Set Status >> Creating Instrument...\nSMO: Init Class\nSMO: Create Instrument\nData: Wait >> 100\nSplash: Set Status >> Creating Instrument UI...\nSMO: Create Instrument UI\nData: Wait >> 100\nSplash: Set Status >> Registering Events...\nEvents: Register\nData: Wait >> 100\nSplash: Set Status >> Starting Instrument...\nSMO: Start Instrument\nData: Wait >> 100\nSplash: Set Status >> Instrument Process Started...\nData: Wait >> 100\nSplash: Set Status >> Starting User Interface...\nSMO: Start Instrument UI\nData: Wait >> 100\nUI: Front Panel State >> Hide\nSMO: Show Instrument UI" ("State(s) in Front (\"\")"), "State(s) in (\"\")"=w363) -> ("States Out"=w362:string)  [unwired: 13 in]
      }
      frame "Macro: Stop SMOs" {
        # "Do not put any code in this frame.\n(It is a separator no-op. You can make a copy of this frame to create a new Macro frame)"
        n132 = call <vilib>:"Add State(s) to Queue__jki_lib_state_machine.vi"("State(s) in Front (\"\")"="UI: Front Panel State >> Show\nSplash: Set Status >> Stopping Instrument...\nSMO: Stop Instrument\nData: Wait >> 100\nSplash: Set Status >> Destroying Instrument...\nSMO: Destroy Instrument\nData: Wait >> 100\nSplash: Set Status >>Hiding UI...\nSMO: Hide Instrument UI\nData: Wait >> 100\nSplash: Set Status >> Stopping UI...\nSMO: Stop Instrument UI\nData: Wait >> 100\nSplash: Set Status >> Destroying UI...\nSMO: Destroy Instrument UI" ("State(s) in Front (\"\")"), "State(s) in (\"\")"=w369) -> ("States Out"=w368:string)  [unwired: 13 in]
      }
      frame "Macro: Exit" {
        # "Exit Macro\n(This is called once, when the VI exits)"
        n133 = Unbundle By Name(w378) -> ("Core.Close Panel on Exit?"=w377:bool)
        n134 = Select(t="UI: Front Panel State >> Open", s=w377, f="") -> (s? t:f=w374:string)
        n135 = call <vilib>:"Add State(s) to Queue__jki_lib_state_machine.vi"("State(s) in Front (\"\")"="UI: Front Panel State >> Open\nUI: Write UI Config\nUI: Exit", "State(s) in (\"\")"=w374, "State(s) at Back (\"\")"="Macro: Stop SMOs\nData: Cleanup\nEvents: Unregister\nExit") -> ("States Out"=w373:string)  [unwired: 12 in]
        n136 = call <vilib>:"Add State(s) to Queue__jki_lib_state_machine.vi"("State(s) in Front (\"\")"=w373, "State(s) in (\"\")"=w381) -> ("States Out"=w380:string)  [unwired: 13 in]
      }
      frame "---------- SMO ----------" {
        # "Do not put any code in this frame.\n(It is a separator no-op. You can make a copy of this frame to create a new Macro frame)"
        n137 = call <vilib>:"Add State(s) to Queue__jki_lib_state_machine.vi"("State(s) in (\"\")"=w386) -> ("States Out"=w385:string)  [unwired: 14 in]
      }
      frame "SMO: Init Class" {
        # "Do not put any code in this frame.\n(It is a separator no-op. You can make a copy of this frame to create a new Macro frame)"
        n138 = Unbundle By Name(w389) -> ("Instrument"=w390:refnum<class "Instrument.lvclass">)
        n139 = case shown="\"Thorlabs\"" "Choose hardware type" {
          tunnel: w390 -> [w396 _ _]
          tunnel: [w396 w397 w398] -> w387
          frame "Simulate", Default {
          }
          frame "PCsensor" {
            w397 = refnum<class "Temperhum.PCSensor.lvclass"> refnum  # Temperhum.PCSensor.lvclass
          }
          frame "Thorlabs" {
            w398 = refnum<class "Temperhum.Thorlabs.lvclass"> refnum  # Temperhum.Thorlabs.lvclass
          }
        }
        n140 = Bundle By Name(cluster=w389, "Instrument"=w387) -> (w388:T6)
        n141 = call <vilib>:"Add State(s) to Queue__jki_lib_state_machine.vi"("State(s) in (\"\")"=w395) -> ("States Out"=w394:string)  [unwired: 14 in]
      }
      frame "SMO: Create Instrument" {
        # "Do not put any code in this frame.\n(It is a separator no-op. You can make a copy of this frame to create a new Macro frame)"
        n142 = Unbundle By Name(w402) -> ("Instrument"=w399:refnum<class "Instrument.lvclass">)
        n143 = call-dynamic "Create Instrument SMO.vi"("error in (no error)"=w406, "Debug Mode? [F]"="Debug Mode", "Configuration Window? [T]"="Config Window", "Instrument in"=w399) -> ("error out"=w405:errorcluster, "Instrument out"=w403:refnum<class "Instrument.lvclass">)  [unwired: 6 in]
        n144 = Bundle By Name(cluster=w402, "Instrument"=w403) -> (w404:T6)
        n145 = call <vilib>:"Add State(s) to Queue__jki_lib_state_machine.vi"("State(s) in (\"\")"=w409) -> ("States Out"=w408:string)  [unwired: 14 in]
      }
      frame "SMO: Start Instrument" {
        # "Do not put any code in this frame.\n(It is a separator no-op. You can make a copy of this frame to create a new Macro frame)"
        n146 = Unbundle By Name(w414) -> ("Instrument"=w415:refnum<class "Instrument.lvclass">)
        n147 = call <vilib>:"Start.vi"("error in (no error)"=w411, "SMO"=w415) -> ("error out"=w410:errorcluster, "SMO out"=w412:refnum<class "Instrument.lvclass">)  [unwired: 8 in]
        n148 = Bundle By Name(cluster=w414, "Instrument"=w412) -> (w413:T6)
        n149 = call <vilib>:"Add State(s) to Queue__jki_lib_state_machine.vi"("State(s) in (\"\")"=w418) -> ("States Out"=w417:string)  [unwired: 14 in]
      }
      frame "SMO: Create Instrument UI" {
        # "Do not put any code in this frame.\n(It is a separator no-op. You can make a copy of this frame to create a new Macro frame)"
        n150 = Unbundle By Name(w425) -> ("Instrument UI"=w423:refnum<class "Instrument UI.lvclass">, "Instrument"=w422:refnum<class "Instrument.lvclass">)
        n151 = call <userlib>:"Create UI.vi"("error in (no error)"=w420, "Instrument in"=w422, "Instrument UI"=w423) -> ("error out"=w419:errorcluster, "Instrument UI out"=w421:refnum<class "Instrument UI.lvclass">)  [unwired: 7 in]
        n152 = Bundle By Name(cluster=w425, "Instrument UI"=w421) -> (w424:T6)
        n153 = call <vilib>:"Add State(s) to Queue__jki_lib_state_machine.vi"("State(s) in (\"\")"=w428) -> ("States Out"=w427:string)  [unwired: 14 in]
      }
      frame "SMO: Start Instrument UI" {
        # "Do not put any code in this frame.\n(It is a separator no-op. You can make a copy of this frame to create a new Macro frame)"
        n154 = Unbundle By Name(w432) -> ("Instrument UI"=w431:refnum<class "Instrument UI.lvclass">)
        n155 = call <vilib>:"Start.vi"("error in (no error)"=w430, "SMO"=w431) -> ("error out"=w429:errorcluster)  [unwired: 8 in, 1 out]
        n156 = call <vilib>:"Add State(s) to Queue__jki_lib_state_machine.vi"("State(s) in (\"\")"=w435) -> ("States Out"=w434:string)  [unwired: 14 in]
      }
      frame "SMO: Show Instrument UI" {
        # "Do not put any code in this frame.\n(It is a separator no-op. You can make a copy of this frame to create a new Macro frame)"
        n157 = Unbundle By Name(w443) -> ("Instrument UI"=w441:refnum<class "Instrument UI.lvclass">)
        n158 = call <vilib>:"GetState.vi"("error in (no error)"=w439, "SMO"=w441) -> ("error out"=w437:errorcluster, "SMO State"=w436:T2, "SMO out"=w440:refnum<class "Instrument UI.lvclass">)  [unwired: 7 in]
        n159 = call <vilib>:"Clear Errors.vi"("error in (no error)"=w437) -> ("error out"=w438:errorcluster)  [unwired: 5 in, 1 out]
        n160 = case shown="\"Started\"" w436 {
          tunnel: [w447 w450] -> w442
          tunnel: w440 -> [_ w449]
          tunnel: w438 -> [w447 w448]
          frame Default {
          }
          frame "Started" {
            n161 = call <vilib>:"Show.vi"("error in (no error)"=w448, "SMO.UI"=w449) -> ("error out"=w450:errorcluster)  [unwired: 8 in, 1 out]
          }
        }
        n162 = call <vilib>:"Add State(s) to Queue__jki_lib_state_machine.vi"("State(s) in (\"\")"=w446) -> ("States Out"=w445:string)  [unwired: 14 in]
      }
      frame "SMO: Destroy Instrument" {
        # "Do not put any code in this frame.\n(It is a separator no-op. You can make a copy of this frame to create a new Macro frame)"
        n163 = Unbundle By Name(w458) -> ("Instrument"=w456:refnum<class "Instrument.lvclass">)
        n164 = call <vilib>:"GetState.vi"("error in (no error)"=w453, "SMO"=w456) -> ("error out"=w452:errorcluster, "SMO State"=w455:T2, "SMO out"=w451:refnum<class "Instrument.lvclass">)  [unwired: 7 in]
        n165 = call <vilib>:"Clear Errors.vi"("error in (no error)"=w452) -> ("error out"=w454:errorcluster)  [unwired: 5 in, 1 out]
        n166 = case shown="\"Stopped\"" w455 {
          tunnel: [w462 w465] -> w457
          tunnel: w454 -> [w462 w464]
          tunnel: w451 -> [_ w463]
          frame Default {
          }
          frame "Stopped" {
            n167 = call <vilib>:"Destroy.vi"("error in (no error)"=w464, "SMO"=w463) -> ("error out"=w465:errorcluster)  [unwired: 9 in]
          }
        }
        n168 = call <vilib>:"Add State(s) to Queue__jki_lib_state_machine.vi"("State(s) in (\"\")"=w461) -> ("States Out"=w460:string)  [unwired: 14 in]
      }
      frame "SMO: Hide Instrument UI" {
        # "Do not put any code in this frame.\n(It is a separator no-op. You can make a copy of this frame to create a new Macro frame)"
        n169 = Unbundle By Name(w473) -> ("Instrument UI"=w471:refnum<class "Instrument UI.lvclass">)
        n170 = call <vilib>:"GetState.vi"("error in (no error)"=w469, "SMO"=w471) -> ("error out"=w467:errorcluster, "SMO State"=w466:T2, "SMO out"=w470:refnum<class "Instrument UI.lvclass">)  [unwired: 7 in]
        n171 = call <vilib>:"Clear Errors.vi"("error in (no error)"=w467) -> ("error out"=w468:errorcluster)  [unwired: 5 in, 1 out]
        n172 = case shown="Default" w466 {
          tunnel: [w477 w480] -> w472
          tunnel: w470 -> [_ w479]
          tunnel: w468 -> [w477 w478]
          frame Default {
          }
          frame "Started" {
            n173 = call <vilib>:"Hide.vi"("error in (no error)"=w478, "SMO.UI"=w479) -> ("error out"=w480:errorcluster)  [unwired: 8 in, 1 out]
          }
        }
        n174 = call <vilib>:"Add State(s) to Queue__jki_lib_state_machine.vi"("State(s) in (\"\")"=w476) -> ("States Out"=w475:string)  [unwired: 14 in]
      }
      frame "SMO: Stop Instrument UI" {
        # "Do not put any code in this frame.\n(It is a separator no-op. You can make a copy of this frame to create a new Macro frame)"
        n175 = Unbundle By Name(w487) -> ("Instrument UI"=w482:refnum<class "Instrument UI.lvclass">)
        n176 = call <vilib>:"GetState.vi"("error in (no error)"=w486, "SMO"=w482) -> ("error out"=w485:errorcluster, "SMO State"=w483:T2, "SMO out"=w481:refnum<class "Instrument UI.lvclass">)  [unwired: 7 in]
        n177 = call <vilib>:"Clear Errors.vi"("error in (no error)"=w485) -> ("error out"=w484:errorcluster)  [unwired: 5 in, 1 out]
        n178 = case shown="\"Created\", \"Started\"" w483 {
          tunnel: [w492 w495] -> w488
          tunnel: w481 -> [_ w494]
          tunnel: w484 -> [w492 w493]
          frame Default {
          }
          frame "Created", "Started" {
            n179 = call <vilib>:"Stop.vi"("error in (no error)"=w493, "SMO"=w494) -> ("error out"=w495:errorcluster)  [unwired: 8 in, 1 out]
          }
        }
        n180 = call <vilib>:"Add State(s) to Queue__jki_lib_state_machine.vi"("State(s) in (\"\")"=w491) -> ("States Out"=w490:string)  [unwired: 14 in]
      }
      frame "SMO: Stop Instrument" {
        # "Do not put any code in this frame.\n(It is a separator no-op. You can make a copy of this frame to create a new Macro frame)"
        n181 = Unbundle By Name(w502) -> ("Instrument"=w497:refnum<class "Instrument.lvclass">)
        n182 = call <vilib>:"GetState.vi"("error in (no error)"=w501, "SMO"=w497) -> ("error out"=w500:errorcluster, "SMO State"=w498:T2, "SMO out"=w496:refnum<class "Instrument.lvclass">)  [unwired: 7 in]
        n183 = call <vilib>:"Clear Errors.vi"("error in (no error)"=w500) -> ("error out"=w499:errorcluster)  [unwired: 5 in, 1 out]
        n184 = case shown="\"Created\", \"Started\"" w498 {
          tunnel: [w507 w510] -> w503
          tunnel: w496 -> [_ w509]
          tunnel: w499 -> [w507 w508]
          frame Default {
          }
          frame "Created", "Started" {
            n185 = call <vilib>:"Stop.vi"("error in (no error)"=w508, "SMO"=w509) -> ("error out"=w510:errorcluster)  [unwired: 8 in, 1 out]
          }
        }
        n186 = call <vilib>:"Add State(s) to Queue__jki_lib_state_machine.vi"("State(s) in (\"\")"=w506) -> ("States Out"=w505:string)  [unwired: 14 in]
      }
      frame "SMO: Destroy Instrument UI" {
        # "Do not put any code in this frame.\n(It is a separator no-op. You can make a copy of this frame to create a new Macro frame)"
        n187 = Unbundle By Name(w517) -> ("Instrument UI"=w516:refnum<class "Instrument UI.lvclass">)
        n188 = call <vilib>:"GetState.vi"("error in (no error)"=w514, "SMO"=w516) -> ("error out"=w513:errorcluster, "SMO State"=w511:T2, "SMO out"=w515:refnum<class "Instrument UI.lvclass">)  [unwired: 7 in]
        n189 = call <vilib>:"Clear Errors.vi"("error in (no error)"=w513) -> ("error out"=w512:errorcluster)  [unwired: 5 in, 1 out]
        n190 = case shown="Default" w511 {
          tunnel: w512 -> [w522 w525]
          tunnel: [w522 w524] -> w518
          tunnel: w515 -> [_ w523]
          frame Default {
          }
          frame "Stopped" {
            n191 = call <vilib>:"Destroy.vi"("error in (no error)"=w525, "SMO"=w523) -> ("error out"=w524:errorcluster)  [unwired: 9 in]
          }
        }
        n192 = call <vilib>:"Add State(s) to Queue__jki_lib_state_machine.vi"("State(s) in (\"\")"=w521) -> ("States Out"=w520:string)  [unwired: 14 in]
      }
      frame "---------- Splash ----------" {
        # "Template Separator\n(You can make a copy of, or modify, this frame)"
        n193 = call <vilib>:"Add State(s) to Queue__jki_lib_state_machine.vi"("State(s) in (\"\")"=w530) -> ("States Out"=w529:string)  [unwired: 14 in]
      }
      frame "Splash: Set Status" {
        # "Your code here.\n(You can make a copy of, or modify, this frame)"
        n194 = property on="Splash Status" class="Str"(error in=w533, "Value"=w534) -> (error out=w532:errorcluster)  [unwired: 1 in, 1 out]
        n195 = call <vilib>:"Add State(s) to Queue__jki_lib_state_machine.vi"("State(s) in (\"\")"=w537) -> ("States Out"=w536:string)  [unwired: 14 in]
      }
      frame "Splash: 2" {
        # "Your code here.\n(You can make a copy of, or modify, this frame)"
        n196 = call <vilib>:"Add State(s) to Queue__jki_lib_state_machine.vi"("State(s) in (\"\")"=w542) -> ("States Out"=w541:string)  [unwired: 14 in]
      }
    }
  }
  "error out" <- w2
